vi "tm421_polling.vi"() -> ()   [LabVIEW 2011]
panel:
  out "Counter":i32
  out "Image":u16[][](graph)
  out "Frames Per Second":dbl
  in  "Quit":bool
  out "Error Out":errorcluster
  # "This is an example of how to check\nfor a new frame instead of waiting\nfor a new frame.  The counter will\nupdate while waiting for a new\nframe to arrive."
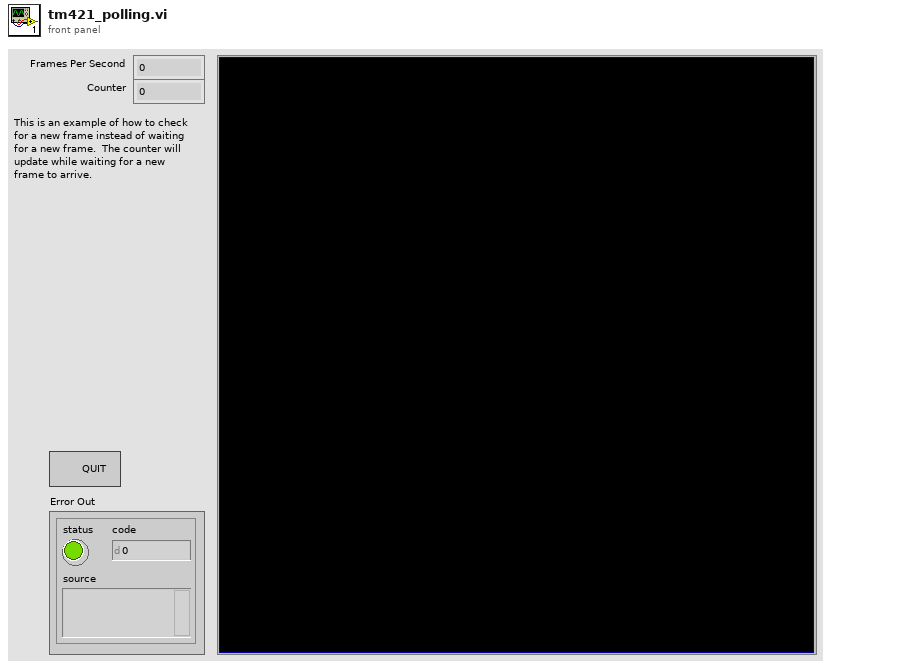
[diagram p1: front panel]
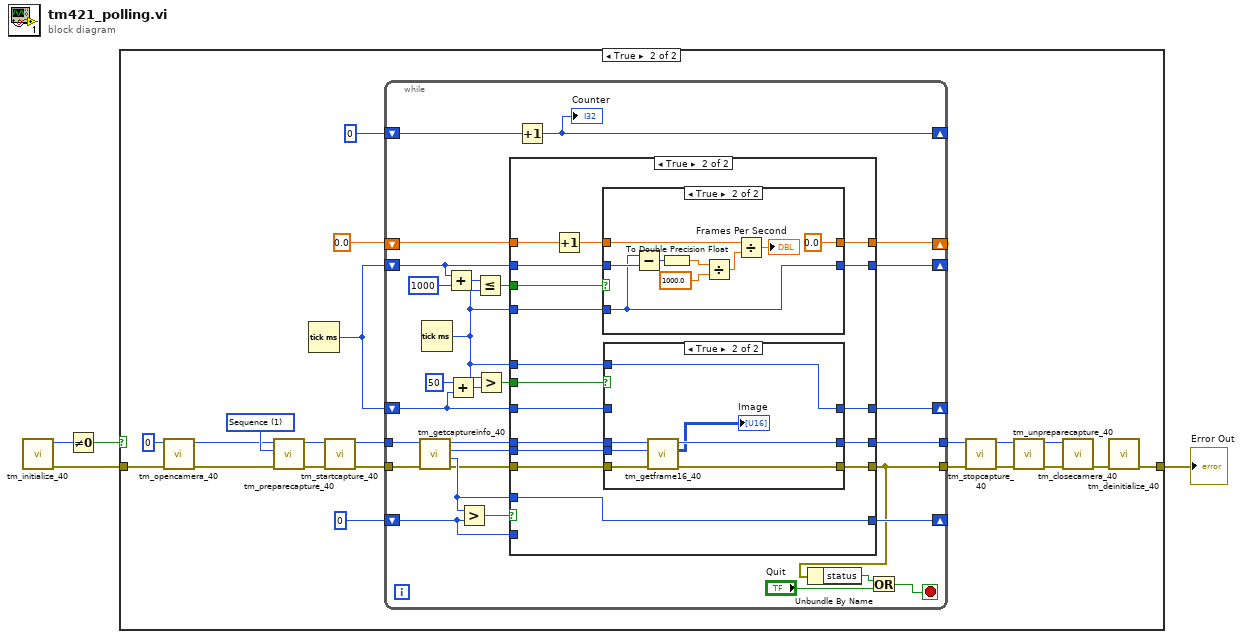
[diagram p0: block diagram]
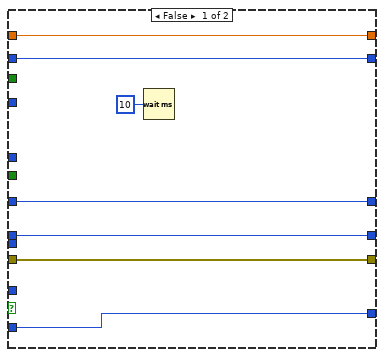
[diagram p3: hidden frame]
diagram:
  n1 = call <userlib>:"tm_initialize_40.vi"() -> ("error out"=w1:errorcluster, "Number Of Cameras"=w2:u32)  [unwired: 8 in, 2 out]
  n2 = Not Equal To 0?(x=w2) -> (x != 0?=w4:bool)
  n3 = case shown="True" w4 {
    tunnel: w1 -> [w5 w26]
    tunnel: [w5 w22] -> w3
    frame False {
    }
    frame True {
      w24 = 1 items=["Snap", "Sequence"] ("Capture mode")
      n4 = call <userlib>:"tm_opencamera_40.vi"("error in (no error)"=w26, "Camera Index"=u32 0) -> ("error out"=w6:errorcluster, "Handle out"=w7:u32)  [unwired: 7 in, 1 out]
      n5 = call <userlib>:"tm_preparecapture_40.vi"("error in (no error)"=w6, "Capture mode"=w24, "Handle in"=w7) -> ("error out"=w15:errorcluster, "Handle out"=w14:u32)  [unwired: 5 in, 2 out]
      n6 = Tick Count (ms)() -> (millisecond timer value=w10:u32)
      n7 = call <userlib>:"tm_startcapture_40.vi"("error in (no error)"=w15, "Handle in"=w14) -> ("error out"=w12:errorcluster, "Handle out"=w13:u32)  [unwired: 8 in]
      n8 = while {
        tunnel: [w44] -> w18
        tunnel: [w43] -> w19
        tunnel: w13 -> [w51]
        tunnel: w12 -> [w50]
        shift-right: [w49] -> _
        shift-left: 0 -> [w48]
        shift-right: [w41] -> _
        shift-left: w10 -> [w29]
        shift-right: [w42] -> _
        shift-left: w10 -> [w30]
        shift-right: [w39] -> _
        shift-left: 0.0 -> [w40]
        shift-right: [w27] -> _
        shift-left: 0 -> [w28]
        stop <- w38 stop-if-true
        n9 = call <userlib>:"tm_getcaptureinfo_40.vi"("error in (no error)"=w50, "Handle in"=w51) -> ("error out"=w46:errorcluster, "Frame Count"=w52:i32, "Frame Index"=w45:i32, "Handle out"=w47:u32)  [unwired: 6 in]
        n10 = Tick Count (ms)() -> (millisecond timer value=w33:u32)
        n11 = Add(x=w29, y=u32 1000) -> (x+y=w34:u32)
        n12 = Add(x=u32 50, y=w30) -> (x+y=w37:u32)
        n13 = Greater?(x=w52, y=w48) -> (0:w53:bool)
        n14 = Less Or Equal?(x=w34, y=w33) -> (x <= y?=w31:bool)
        n15 = Greater?(x=w33, y=w37) -> (0:w32:bool)
        n16 = case shown="True" w53 {
          tunnel: w48 -> [w62 _]
          tunnel: [w62 w65] -> w49
          tunnel: w52 -> [_ w65]
          tunnel: w47 -> [w60 w79]
          tunnel: w46 -> [w61 w77]
          tunnel: w45 -> [_ w78]
          tunnel: [w61 w73] -> w43
          tunnel: [w60 w74] -> w44
          tunnel: w29 -> [w58 w76]
          tunnel: w30 -> [w59 w75]
          tunnel: [w59 w72] -> w42
          tunnel: [w58 w71] -> w41
          tunnel: w40 -> [w57 w63]
          tunnel: [w57 w70] -> w39
          tunnel: w33 -> [_ w69]
          tunnel: w33 -> [_ w68]
          tunnel: w32 -> [_ w67]
          tunnel: w31 -> [_ w66]
          frame False {
            n17 = Wait (ms)(milliseconds to wait=u32 10) -> ()  [unwired: 1 out]
          }
          frame True {
            n18 = Increment(x=w63) -> (x+1=w64:dbl)
            n19 = case shown="True" w66 {
              tunnel: w76 -> [w91 w94]
              tunnel: [w91 w92] -> w71
              tunnel: w64 -> [w90 w98]
              tunnel: w69 -> [_ w92]
              tunnel: [w90 0.0] -> w70
              frame False {
              }
              frame True {
                n20 = Subtract(x=w92, y=w94) -> (x-y=w93:u32)
                n21 = To Double Precision Float(number=w93) -> (double precision float=w100:dbl)
                n22 = Divide(x=w100, y=1000.0) -> (x/y=w97:dbl)
                n23 = Divide(x=w98, y=w97) -> (x/y=→"Frames Per Second":dbl)
              }
            }
            n24 = case shown="True" w67 {
              tunnel: w79 -> [w82 w89]
              tunnel: w77 -> [w81 w88]
              tunnel: w78 -> [_ w87]
              tunnel: w75 -> [w80 _]
              tunnel: w68 -> [_ w86]
              tunnel: [w82 w84] -> w74
              tunnel: [w81 w85] -> w73
              tunnel: [w80 w86] -> w72
              frame False {
              }
              frame True {
                n25 = call <userlib>:"tm_getframe16_40.vi"("error in (no error)"=w88, "Frame Index"=w87, "Handle in"=w89) -> ("error out"=w85:errorcluster, "Data"=→"Image":u16[][], "Handle out"=w84:u32)  [unwired: 5 in, 1 out]
              }
            }
          }
        }
        n26 = Increment(x=w28) -> (x+1=w27:i32)
        "Counter" <- w27
        n27 = Unbundle By Name(w43) -> ("status"=w55:bool)
        n28 = Or(x=w55, y="Quit") -> (x .or. y?=w38:bool)
      }
      n29 = call <userlib>:"tm_stopcapture_40.vi"("error in (no error)"=w19, "Handle in"=w18) -> ("error out"=w16:errorcluster, "Handle out"=w17:u32)  [unwired: 8 in]
      n30 = call <userlib>:"tm_unpreparecapture_40.vi"("error in (no error)"=w16, "Handle in"=w17) -> ("error out"=w21:errorcluster, "Handle out"=w20:u32)  [unwired: 8 in]
      n31 = call <userlib>:"tm_closecamera_40.vi"("error in (no error)"=w21, "Handle in"=w20) -> ("error out"=w23:errorcluster)  [unwired: 9 in]
      n32 = call <userlib>:"tm_deinitialize_40.vi"("error in (no error)"=w23) -> ("error out"=w22:errorcluster)  [unwired: 10 in]
    }
  }
  "Error Out" <- w3
